vi "_caraya_updatePPLbuildspec.vi"(8 "error in (no error)":errorcluster, 10 "Version":string, 11 "Project Path":path=path "C:/Projects/JKI/Caraya/src/tests/test-all-asserts/Test Runner.AllAsserts.lvclass") -> (0 "error out":errorcluster)   [LabVIEW 2013]
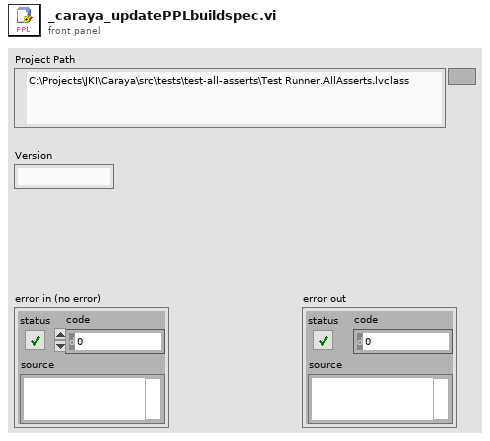
[diagram p1: front panel]
types:
  T1 = enum16{"open", "replace", "create", "open or create", "replace or create", "replace or create with confirmation"}
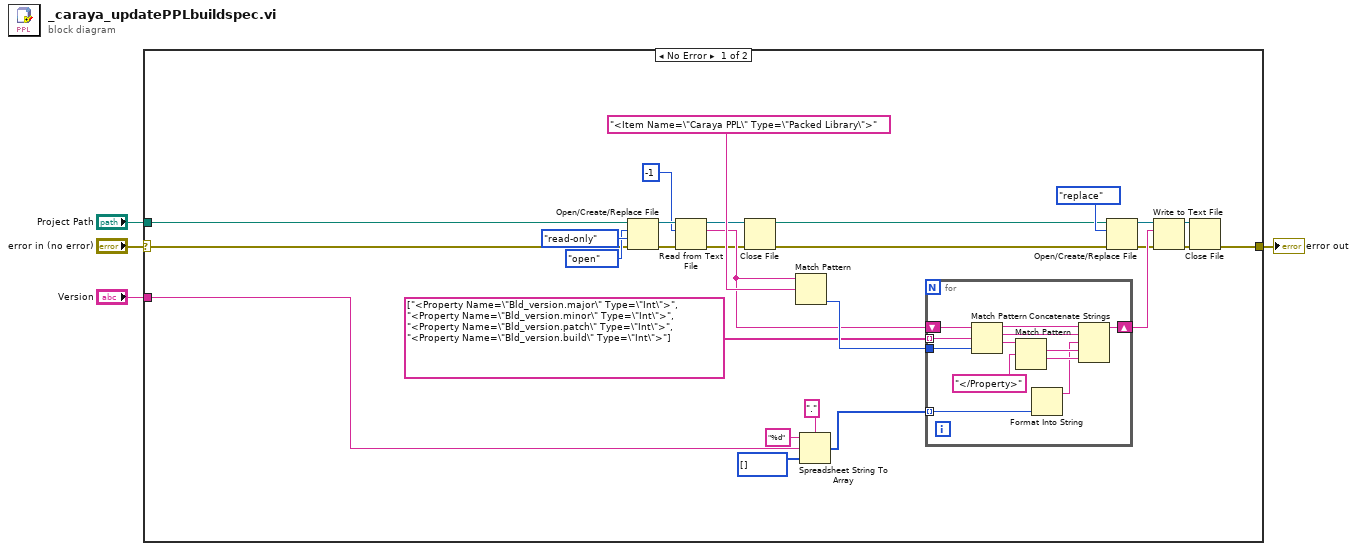
[diagram p0: block diagram]
diagram:
  n1 = case shown="No Error" "error in (no error)" {
    selector: "error in (no error)" -> [w8 w44]
    tunnel: "Project Path" -> [w6 _]
    tunnel: [w7 w44] -> w3
    tunnel: "Version" -> [w5 _]
    frame No Error {
      n2 = Open/Create/Replace File(file path (use dialog)=w6, error in=w8, operation (0:open)=T1."open", access (0:read/write)=enum16{"read/write", "read-only", "write-only"}."read-only") -> (refnum out=w29:refnum<file>, error out=w30:errorcluster)  [unwired: 2 in, 1 out]
      n3 = Read from Text File(file (use dialog)=w29, count=-1, error in=w30) -> (refnum out=w20:refnum<file>, text=w21:string, error out=w19:errorcluster)  [unwired: 1 in, 1 out]
      n4 = Close File(refnum=w20, error in=w19) -> (path=w15:path, error out=w18:errorcluster)
      n5 = Match Pattern(string=w21, regular expression="<Item Name=\"Caraya PPL\" Type=\"Packed Library\">") -> (offset past match=w23:i32)  [unwired: 1 in, 3 out]
      n6 = Spreadsheet String To Array(delimiter (Tab)=".", format string="%d", spreadsheet string=w5, array type (2D Dbl)=u16[] []) -> (array=w9:u16[])
      n7 = for {
        tunnel: string[] ["<Property Name=\"Bld_version.major\" Type=\"Int\">", "<Property Name=\"Bld_version.minor\" Type=\"Int\">", "<Property Name=\"Bld_version.patch\" Type=\"Int\">", "<Property Name=\"Bld_version.build\" Type=\"Int\">"] -> [w43] mode=indexing
        tunnel: w23 -> [w36]
        shift-right: [w37] -> w31
        shift-left: w21 -> [w35]
        tunnel: w9 -> [w32] mode=indexing
        n8 = Match Pattern(string=w35, regular expression=w43, offset (0)=w36) -> (before substring=w41:string, match substring=w40:string, after substring=w42:string)  [unwired: 1 out]
        n9 = Match Pattern(string=w42, regular expression="</Property>") -> (match substring=w39:string, after substring=w38:string)  [unwired: 1 in, 2 out]
        n10 = Format Into String(w32) -> (resulting string=w33:string)  [unwired: 3 in, 1 out]
        n11 = Concatenate Strings(w41, w40, w33, w39, w38) -> (w37:string)
      }
      n12 = Open/Create/Replace File(file path (use dialog)=w15, error in=w18, operation (0:open)=T1."replace") -> (refnum out=w14:refnum<file>, error out=w17:errorcluster)  [unwired: 3 in, 1 out]
      n13 = Write to Text File(file (use dialog)=w14, text=w31, error in=w17) -> (refnum out=w25:refnum<file>, error out=w26:errorcluster)  [unwired: 1 in, 1 out]
      n14 = Close File(refnum=w25, error in=w26) -> (error out=w7:errorcluster)  [unwired: 1 out]
    }
    frame Error {
    }
  }
  "error out" <- w3
